vi "MerweScSigPts_GetNumSigmas.vi"(11 "MerweScaledSigmaPts":T1) -> (3 "NumSigmas":i32)   [LabVIEW 2019, in "Trajectory_Library.lvlib"]
doc: "Returns number of sigma points for each variable in the state x.\n \n\nInputs:\n - MerweScaledSigmaPts -- data cluster\n\nOutputs:\n - NumSigmas -- The number of sigma points for each variable in the state x."
uses:
  Trajectory_Library.lvlib
  MERWE_SCALED_SIGMA_PTS.ctl
  <vilib>/Analysis/Matrix/Datatypes/RealMatrix.ctl
  <vilib>/Analysis/Matrix/NI_Matrix.lvlib
panel:
  # "<?, 1>"
  # "<?, 1>"
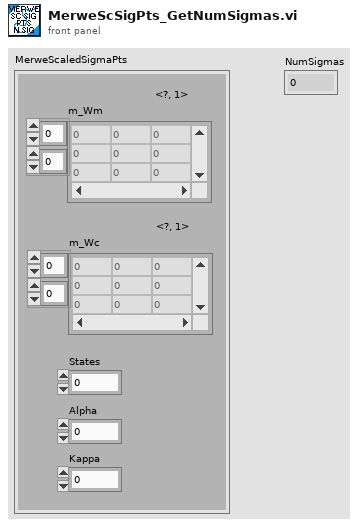
[diagram p1: front panel]
types:
  T1 = typedef "Trajectory_Library.lvlib/MERWE_SCALED_SIGMA_PTS.ctl" = cluster{"m_Wm":T2, "States":i32, "Alpha":dbl, "m_Wc":T2, "Kappa":i32}
  T2 = typedef "NI_Matrix.lvlib/RealMatrix.ctl" = dbl[][]
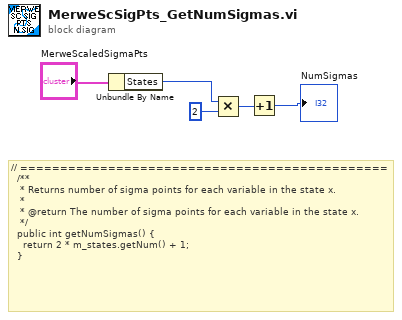
[diagram p0: block diagram]
diagram:
  # "// ==============================================\n  /**\n   * Returns number of sigma points for each variable in the state x.\n   *\n   * @return The number of sigma points for each variable in the state x.\n   */\n  public int getNumSigmas() {\n    return 2 * m_states.getNum() + 1;\n  }"
  n1 = Unbundle By Name("MerweScaledSigmaPts") -> ("States"=w4:i32)
  n2 = Multiply(x=w4, y=2) -> (x*y=w2:i32)
  n3 = Increment(x=w2) -> (x+1=→"NumSigmas":i32)
